vi "Find Digital Pattern Events.vi"(7 "Base.length":dbl, 9 "Event":T1, 10 "Pattern":T2, 11 "Rotations":u16) -> (2 "crank angle":bool, 3 "Locations":dbl[](array[numeric]), 5 "first falling":bool)   [LabVIEW 2019, in "Engine Simulation Toolkit System Explorer.lvlib"]
uses:
  Engine Simulation Toolkit System Explorer.lvlib
  Digital Pattern Expanded.ctl
  Digital Pattern Find Events Enum.ctl
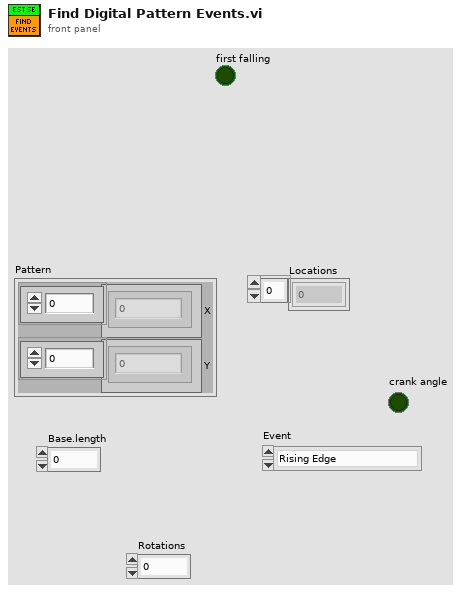
[diagram p1: front panel]
types:
  T1 = typedef "Engine Simulation Toolkit System Explorer.lvlib/Digital Pattern Find Events Enum.ctl" = enum16{"Rising Edge", "Falling Edge", "Any Edge", "Center Tooth", "Center Gap"}
  T2 = typedef "Engine Simulation Toolkit System Explorer.lvlib/Digital Pattern Expanded.ctl" = cluster{"X":dbl[], "Y":dbl[]}
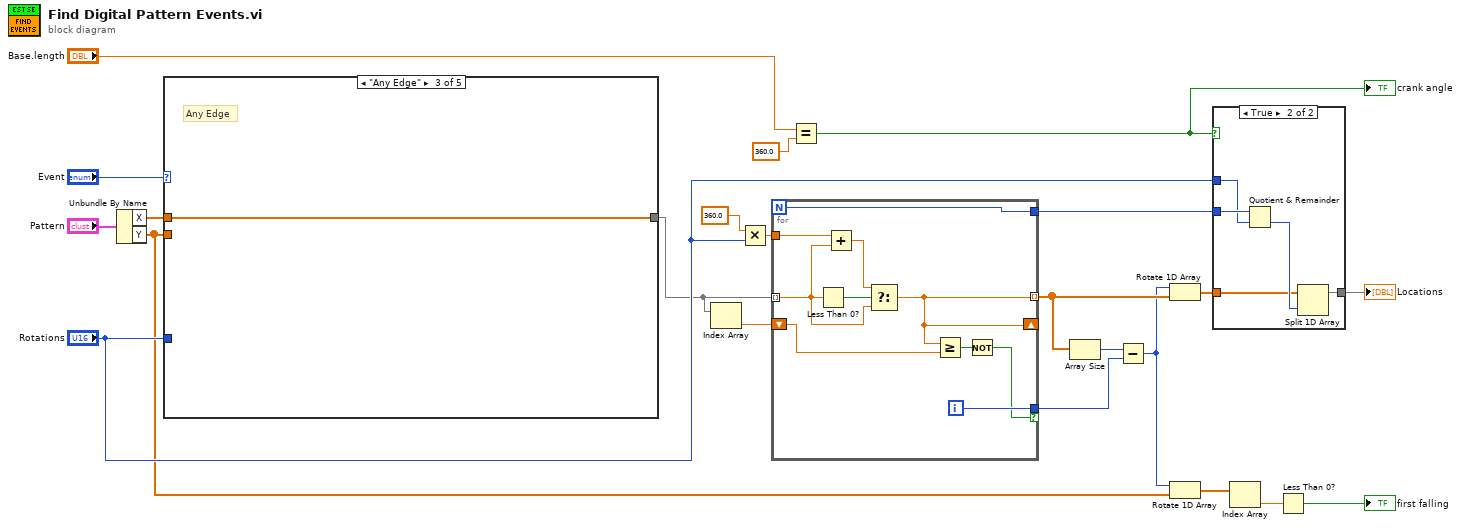
[diagram p0: block diagram]
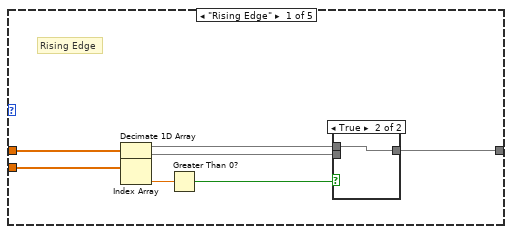
[diagram p3: hidden frame]
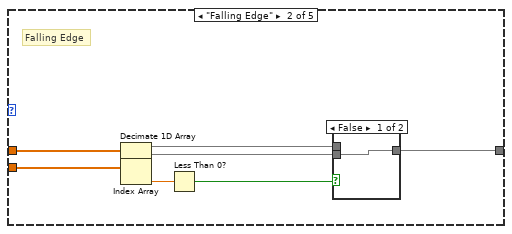
[diagram p5: hidden frame]
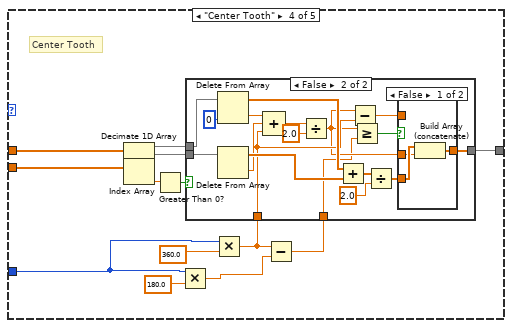
[diagram p7: hidden frame]
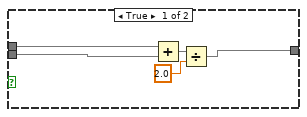
[diagram p8: hidden frame]
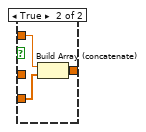
[diagram p9: hidden frame]
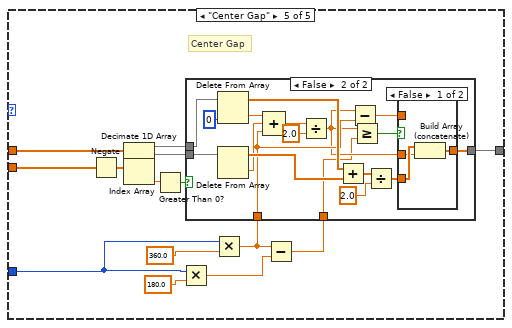
[diagram p10: hidden frame]
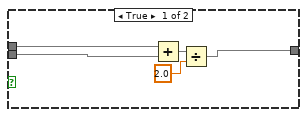
[diagram p11: hidden frame]
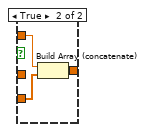
[diagram p12: hidden frame]
diagram:
  n1 = Unbundle By Name("Pattern") -> ("X"=w6:dbl[], "Y"=w4:dbl[])
  n2 = case shown="\"Any Edge\"" "Event" {
    tunnel: "Rotations" -> [_ _ _ w54 w86]
    tunnel: [w29 w38 w41 w52 w95] -> w9
    tunnel: w4 -> [w24 w33 _ w43 w85]
    tunnel: w6 -> [w23 w32 w41 w42 w84]
    frame "Rising Edge" {
      # "Rising Edge"
      n3 = Decimate 1D Array(w23) -> (w26:dbl[], w25:dbl[])
      n4 = Index Array(array=w24) -> (element=w28:dbl)  [unwired: 1 in]
      n5 = Greater Than 0?(x=w28) -> (x > 0?=w27:bool)
      n6 = case shown="True" w27 {
        tunnel: [w30 w31] -> w29
        tunnel: w26 -> [_ w31]
        tunnel: w25 -> [w30 _]
        frame False {
        }
        frame True {
        }
      }
    }
    frame "Falling Edge" {
      # "Falling Edge"
      n7 = Decimate 1D Array(w32) -> (w35:dbl[], w34:dbl[])
      n8 = Index Array(array=w33) -> (element=w37:dbl)  [unwired: 1 in]
      n9 = Less Than 0?(x=w37) -> (x < 0?=w36:bool)
      n10 = case shown="False" w36 {
        tunnel: [w39 w40] -> w38
        tunnel: w35 -> [_ w40]
        tunnel: w34 -> [w39 _]
        frame False {
        }
        frame True {
        }
      }
    }
    frame "Any Edge" {
      # "Any Edge"
    }
    frame "Center Tooth" {
      # "Center Tooth"
      n11 = Decimate 1D Array(w42) -> (w48:dbl[], w47:dbl[])
      n12 = Index Array(array=w43) -> (element=w50:dbl)  [unwired: 1 in]
      n13 = Greater Than 0?(x=w50) -> (x > 0?=w49:bool)
      n14 = Multiply(x=w54, y=180.0 ("t")) -> (x*y=w44:dbl)
      n15 = Multiply(x=w54, y=360.0 ("t")) -> (x*y=w53:dbl)
      n16 = Subtract(x=w53, y=w44) -> (x-y=w51:dbl)
      n17 = case shown="False" w49 {
        tunnel: w48 -> [w59 w76]
        tunnel: w47 -> [w58 w71]
        tunnel: [w55 w62] -> w52
        tunnel: w53 -> [_ w66]
        tunnel: w51 -> [_ w60]
        frame True {
          n18 = Add(x=w59, y=w58) -> (x+y=w57:dbl[])
          n19 = Divide(x=w57, y=2.0) -> (x/y=w55:dbl[])
        }
        frame False {
          n20 = Delete From Array(array=w76, index=0) -> (deleted portion=w75:dbl, array with subset deleted=w69:dbl[])  [unwired: 1 in]
          n21 = Delete From Array(array=w71) -> (deleted portion=w67:dbl, array with subset deleted=w70:dbl[])  [unwired: 2 in]
          n22 = Compound Arithmetic op=ADD(w75, w67, w66) -> (w73:dbl)
          n23 = Divide(x=w73, y=2.0) -> (x/y=w61:dbl)
          n24 = Add(x=w69, y=w70) -> (x+y=w77:dbl[])
          n25 = Subtract(x=w61, y=w66) -> (x-y=w64:dbl)
          n26 = Greater Or Equal?(x=w61, y=w60) -> (x >= y?=w65:bool)
          n27 = Divide(x=w77, y=2.0) -> (x/y=w63:dbl[])
          n28 = case shown="False" w65 {
            tunnel: w64 -> [_ w83]
            tunnel: w63 -> [w79 w82]
            tunnel: [w80 w81] -> w62
            tunnel: w61 -> [w78 _]
            frame False {
              n29 = Build Array (concatenate)(w79, w78) -> (w80:dbl[])
            }
            frame True {
              n30 = Build Array (concatenate)(w83, w82) -> (w81:dbl[])
            }
          }
        }
      }
    }
    frame "Center Gap" {
      # "Center Gap"
      n31 = Negate(x=w85) -> (-x=w87:dbl[])
      n32 = Decimate 1D Array(w84) -> (w89:dbl[], w88:dbl[])
      n33 = Index Array(array=w87) -> (element=w91:dbl)  [unwired: 1 in]
      n34 = Greater Than 0?(x=w91) -> (x > 0?=w90:bool)
      n35 = Multiply(x=w86, y=180.0 ("t")) -> (x*y=w96:dbl)
      n36 = Multiply(x=w86, y=360.0 ("t")) -> (x*y=w97:dbl)
      n37 = Subtract(x=w97, y=w96) -> (x-y=w94:dbl)
      n38 = case shown="False" w90 {
        tunnel: w89 -> [w102 w119]
        tunnel: w88 -> [w101 w114]
        tunnel: [w98 w105] -> w95
        tunnel: w97 -> [_ w109]
        tunnel: w94 -> [_ w103]
        frame True {
          n39 = Add(x=w102, y=w101) -> (x+y=w100:dbl[])
          n40 = Divide(x=w100, y=2.0) -> (x/y=w98:dbl[])
        }
        frame False {
          n41 = Delete From Array(array=w119, index=0) -> (deleted portion=w118:dbl, array with subset deleted=w112:dbl[])  [unwired: 1 in]
          n42 = Delete From Array(array=w114) -> (deleted portion=w110:dbl, array with subset deleted=w113:dbl[])  [unwired: 2 in]
          n43 = Compound Arithmetic op=ADD(w118, w110, w109) -> (w116:dbl)
          n44 = Divide(x=w116, y=2.0) -> (x/y=w104:dbl)
          n45 = Add(x=w112, y=w113) -> (x+y=w120:dbl[])
          n46 = Subtract(x=w104, y=w109) -> (x-y=w107:dbl)
          n47 = Greater Or Equal?(x=w104, y=w103) -> (x >= y?=w108:bool)
          n48 = Divide(x=w120, y=2.0) -> (x/y=w106:dbl[])
          n49 = case shown="False" w108 {
            tunnel: w107 -> [_ w126]
            tunnel: w106 -> [w122 w125]
            tunnel: [w123 w124] -> w105
            tunnel: w104 -> [w121 _]
            frame False {
              n50 = Build Array (concatenate)(w122, w121) -> (w123:dbl[])
            }
            frame True {
              n51 = Build Array (concatenate)(w126, w125) -> (w124:dbl[])
            }
          }
        }
      }
    }
  }
  n52 = Index Array(array=w9) -> (element=w18:dbl)  [unwired: 1 in]
  n53 = Multiply(x=360.0, y="Rotations") -> (x*y=w20:dbl)
  n54 = for {
    N -> [w127]
    tunnel: w9 -> [w134] mode=indexing
    tunnel: [w131] -> w17 mode=indexing
    tunnel: w20 -> [w133]
    tunnel: [w132] -> w15 if=w128
    shift-right: [w131] -> _
    shift-left: w18 -> [w130]
    tunnel: [w127] -> w14
    i -> [w132]
    n55 = Less Than 0?(x=w134) -> (x < 0?=w136:bool)
    n56 = Add(x=w133, y=w134) -> (x+y=w135:dbl)
    n57 = Select(t=w135, s=w136, f=w134) -> (s? t:f=w131:dbl)
    n58 = Greater Or Equal?(x=w131, y=w130) -> (x >= y?=w129:bool)
    n59 = Not(x=w129) -> (.not. x?=w128:bool)
  }
  n60 = Equal?(x="Base.length", y=360.0) -> (x = y?=w12:bool)
  "crank angle" <- w12
  n61 = Array Size(array=w17) -> (size(s)=w16:i32)
  n62 = Subtract(x=w16, y=w15) -> (x-y=w3:i32)
  n63 = Rotate 1D Array(1:w17, 2:w3) -> (0:w13:dbl[])
  n64 = Rotate 1D Array(1:w4, 2:w3) -> (0:w1:dbl[])
  n65 = case shown="True" w12 {
    tunnel: w14 -> [_ w142]
    tunnel: "Rotations" -> [_ w141]
    tunnel: w13 -> [w137 w139]
    tunnel: [w137 w138] -> w8
    frame False {
    }
    frame True {
      n66 = Quotient & Remainder(x=w142, y=w141) -> (floor(x/y)=w140:i32)  [unwired: 1 out]
      n67 = Split 1D Array(array=w139, index=w140) -> (first subarray=w138:dbl[])  [unwired: 1 out]
    }
  }
  "Locations" <- w8
  n68 = Index Array(array=w1) -> (element=w2:dbl)  [unwired: 1 in]
  n69 = Less Than 0?(x=w2) -> (x < 0?=→"first falling":bool)
